vi "Package Peaks and Calculate FP.vi"(3 "peaks data":T1={"maxes"=[0, 0, 0, 0], "sums"=[0, 0, 0, 0], "time inside"=0, "time outside"=0}, 4 "Sort Case":i8(ring)=1 items=["Peak Max", "Peak Average", "Max and Ratio", "Average and Ratio"], 7 "Array 2":cluster{"[0]":i32, "[1]":i32, "[2]":i32}[](array[cluster])=[{"[0]"=3276800, "[1]"=1000, "[2]"=1}, {"[0]"=3276800, "[1]"=1000, "[2]"=1}, {"[0]"=0, "[1]"=0, "[2]"=0}, {"[0]"=0, "[1]"=0, "[2]"=1}], 11 "N1d in":u32, 13 "Sa":i8(ring) items=["PMT1", "PMT2", "PMT3", "PMT4"], 15 "Sb":i8(ring)=1 items=["PMT1", "PMT2", "PMT3", "PMT4"], 17 "sort all":bool, 19 "sort one":bool) -> (18 "sort!":bool, 24 "M1,M2,M3,M4,S1,S2,S3,S4,Tin,Tout,FP,Sort?":i32[](array[numeric]), 27 "N1d out":u32)   [LabVIEW 2009]
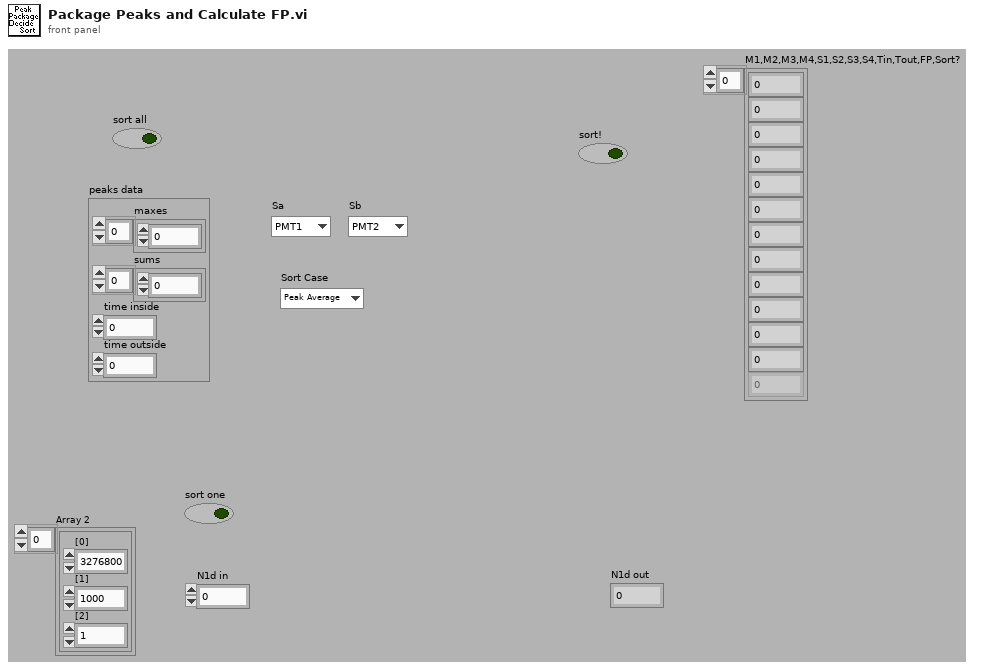
[diagram p1: front panel]
types:
  T1 = cluster{"maxes":i16[], "sums":i32[], "time inside":i32, "time outside":i32}
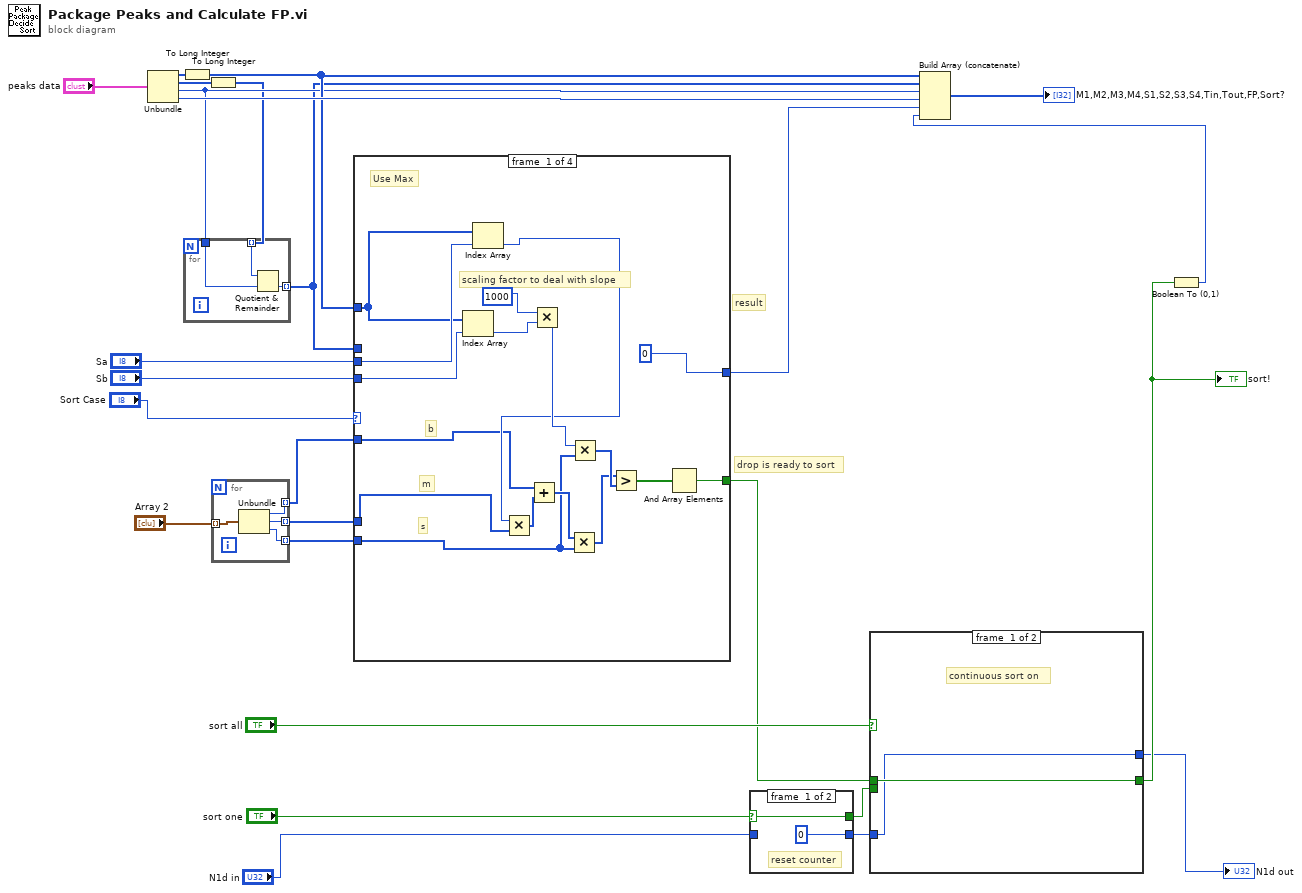
[diagram p0: block diagram]
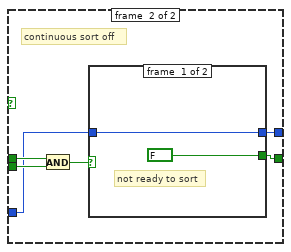
[diagram p2: hidden frame]
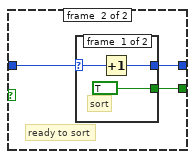
[diagram p3: hidden frame]
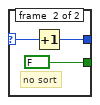
[diagram p4: hidden frame]
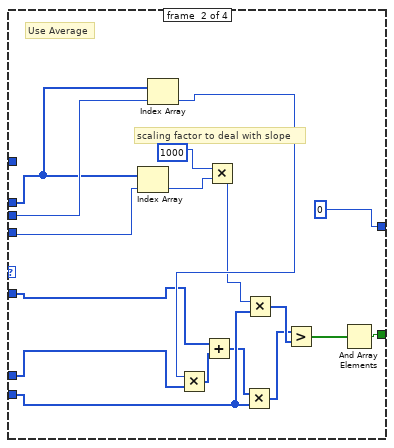
[diagram p6: hidden frame]
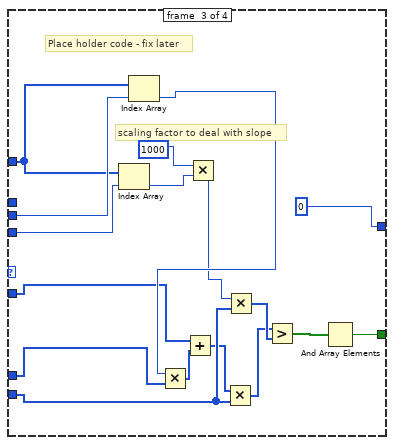
[diagram p7: hidden frame]
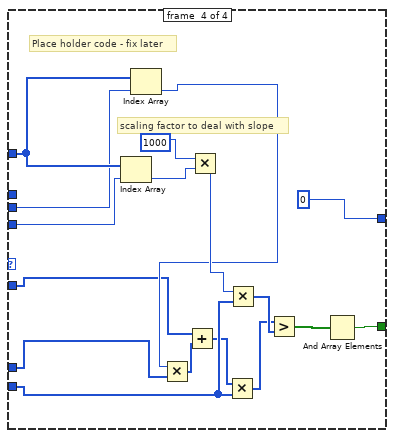
[diagram p8: hidden frame]
diagram:
  # "drop is ready to sort"
  # "result"
  n1 = Unbundle("peaks data") -> ("maxes"=w22:i16[], "sums"=w21:i32[], "time inside"=w17:i32, "time outside"=w24:i32)
  n2 = To Long Integer(number=w22) -> (32bit integer=w20:i32[])
  n3 = To Long Integer(number=w21) -> (32bit integer=w16:i32[])
  n4 = for {
    tunnel: w17 -> [w29]
    tunnel: w16 -> [w28] mode=indexing
    tunnel: [w27] -> w15 mode=indexing
    n5 = Quotient & Remainder(x=w28, y=w29) -> (floor(x/y)=w27:i32)  [unwired: 1 out]
  }
  n6 = for {
    tunnel: "Array 2" -> [w33] mode=indexing
    tunnel: [w32] -> w11 mode=indexing
    tunnel: [w31] -> w10 mode=indexing
    tunnel: [w30] -> w9 mode=indexing
    n7 = Unbundle(w33) -> ("[0]"=w32:i32, "[1]"=w31:i32, "[2]"=w30:i32)
  }
  n8 = case shown="0, Default" "Sort Case" {
    tunnel: "Sa" -> [w50 w64 w81 w94]
    tunnel: "Sb" -> [w48 w63 w80 w93]
    tunnel: [i16 0 i16 0 i16 0 i16 0] -> w18
    tunnel: w20 -> [w49 _ w79 w95]
    tunnel: w15 -> [_ w58 _ _]
    tunnel: [w43 w60 w75 w92] -> w6
    tunnel: w11 -> [w36 w55 w74 w91]
    tunnel: w10 -> [w35 w56 w73 w90]
    tunnel: w9 -> [w34 w57 w72 w89]
    frame #0 {
      # "s"
      # "m"
      # "b"
      # "scaling factor to deal with slope"
      # "Use Max"
      n9 = Index Array(array=w49, index=w48) -> (element=w46:i32)
      n10 = Index Array(array=w49, index=w50) -> (element=w41:i32)
      n11 = Multiply(x=w41, y=w35) -> (x*y=w40:i32[])
      n12 = Add(x=w36, y=w40) -> (x+y=w38:i32[])
      n13 = Multiply(x=1000, y=w46) -> (x*y=w42:i32)
      n14 = Multiply(x=w38, y=w34) -> (x*y=w37:i32[])
      n15 = Multiply(x=w42, y=w34) -> (x*y=w39:i32[])
      n16 = Greater?(x=w37, y=w39) -> (0:w44:bool[])
      n17 = And Array Elements(Boolean array=w44) -> (logical AND=w43:bool)
    }
    frame #1 {
      # "scaling factor to deal with slope"
      # "Use Average"
      n18 = Index Array(array=w58, index=w63) -> (element=w67:i32)
      n19 = Index Array(array=w58, index=w64) -> (element=w62:i32)
      n20 = Multiply(x=w62, y=w56) -> (x*y=w54:i32[])
      n21 = Add(x=w55, y=w54) -> (x+y=w52:i32[])
      n22 = Multiply(x=1000, y=w67) -> (x*y=w59:i32)
      n23 = Multiply(x=w52, y=w57) -> (x*y=w51:i32[])
      n24 = Multiply(x=w59, y=w57) -> (x*y=w53:i32[])
      n25 = Greater?(x=w51, y=w53) -> (0:w65:bool[])
      n26 = And Array Elements(Boolean array=w65) -> (logical AND=w60:bool)
    }
    frame #2 {
      # "Place holder code - fix later"
      # "scaling factor to deal with slope"
      n27 = Index Array(array=w79, index=w80) -> (element=w84:i32)
      n28 = Index Array(array=w79, index=w81) -> (element=w78:i32)
      n29 = Multiply(x=w78, y=w73) -> (x*y=w71:i32[])
      n30 = Add(x=w74, y=w71) -> (x+y=w69:i32[])
      n31 = Multiply(x=1000, y=w84) -> (x*y=w76:i32)
      n32 = Multiply(x=w69, y=w72) -> (x*y=w68:i32[])
      n33 = Multiply(x=w76, y=w72) -> (x*y=w70:i32[])
      n34 = Greater?(x=w68, y=w70) -> (0:w82:bool[])
      n35 = And Array Elements(Boolean array=w82) -> (logical AND=w75:bool)
    }
    frame #3 {
      # "Place holder code - fix later"
      # "scaling factor to deal with slope"
      n36 = Index Array(array=w95, index=w93) -> (element=w101:i32)
      n37 = Index Array(array=w95, index=w94) -> (element=w96:i32)
      n38 = Multiply(x=w96, y=w90) -> (x*y=w88:i32[])
      n39 = Add(x=w91, y=w88) -> (x+y=w86:i32[])
      n40 = Multiply(x=1000, y=w101) -> (x*y=w97:i32)
      n41 = Multiply(x=w86, y=w89) -> (x*y=w85:i32[])
      n42 = Multiply(x=w97, y=w89) -> (x*y=w87:i32[])
      n43 = Greater?(x=w85, y=w87) -> (0:w99:bool[])
      n44 = And Array Elements(Boolean array=w99) -> (logical AND=w92:bool)
    }
  }
  n45 = case shown="True" "sort one" {
    selector: "sort one" -> [w103 w105]
    tunnel: [w103 w105] -> w4
    tunnel: [u32 0 ("N1d") w104] -> w2
    tunnel: "N1d in" -> [_ w104]
    frame #0 {
      # "reset counter"
    }
    frame #1 {
    }
  }
  n46 = case shown="False" "sort all" {
    tunnel: w4 -> [_ w113]
    tunnel: w6 -> [w107 w112]
    tunnel: [w107 w111] -> w8
    tunnel: w2 -> [w106 w109]
    tunnel: [w106 w108] -> w1
    frame #0 {
      # "continuous sort on"
    }
    frame #1 {
      # "continuous sort off"
      n47 = And(x=w112, y=w113) -> (x .and. y?=w110:bool)
      n48 = case shown="True" w110 {
        tunnel: [FALSE w118] -> w111
        tunnel: w109 -> [w114 w117]
        tunnel: [w114 w116] -> w108
        frame #0 {
          # "not ready to sort"
        }
        frame #1 {
          # "ready to sort"
          n49 = case shown="Default" w117 {
            selector: w117 -> [w120 w123]
            tunnel: [TRUE FALSE] -> w118
            tunnel: [w119 w122] -> w116
            frame #0 {
              # "sort"
              n50 = Increment(x=w120) -> (x+1=w119:u32)
            }
            frame #1 {
              # "no sort"
              n51 = Increment(x=w123) -> (x+1=w122:u32)
            }
          }
        }
      }
    }
  }
  "sort!" <- w8
  "N1d out" <- w1
  n52 = Boolean To (0,1)(Boolean=w8) -> (0, 1=w23:i16)
  n53 = Build Array (concatenate)(w20, w15, w17, w24, w18, w23) -> (→"M1,M2,M3,M4,S1,S2,S3,S4,Tin,Tout,FP,Sort?":i32[])
